vi "MULTTCP_CB_findcmd.vi"(9 "pending in":T1[](array[typedef]), 10 "message":string, 11 "cmds":string[](array[string])) -> (1 "pending out":T1[](array[typedef]), 2 "found":bool, 6 "cmd index":i32)   [LabVIEW 2016]
uses:
  MULTTCP_BlockingStruct.ctl
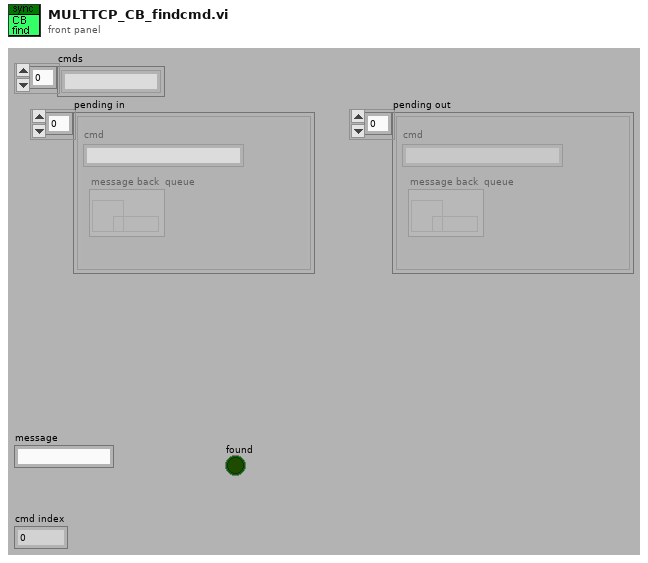
[diagram p1: front panel]
types:
  T1 = typedef "MULTTCP_BlockingStruct.ctl" = cluster{"cmd":string, "message back  queue":refnum<queue>}
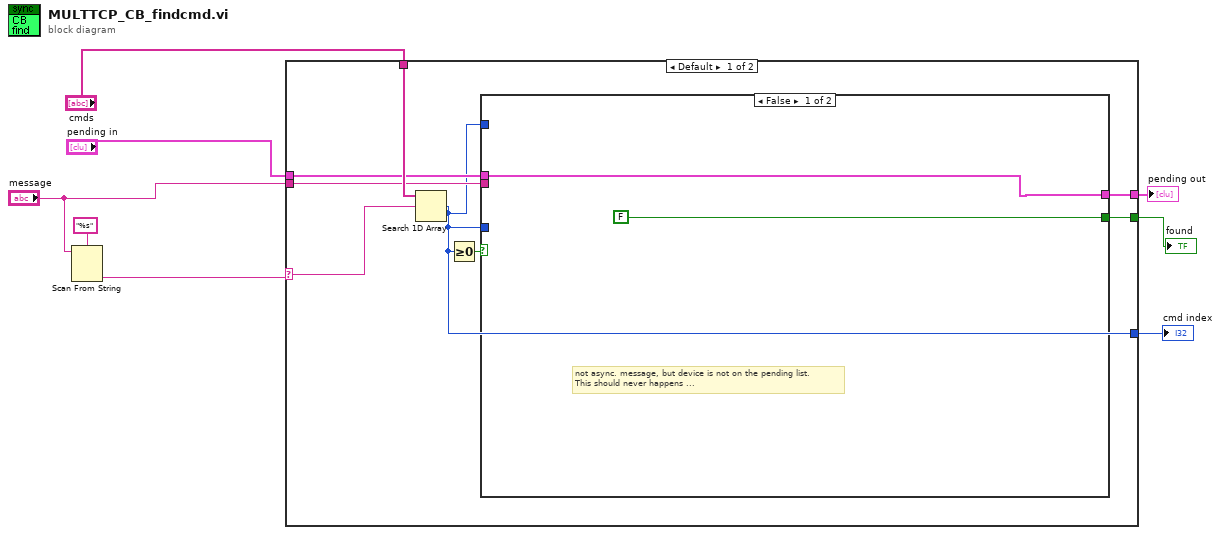
[diagram p0: block diagram]
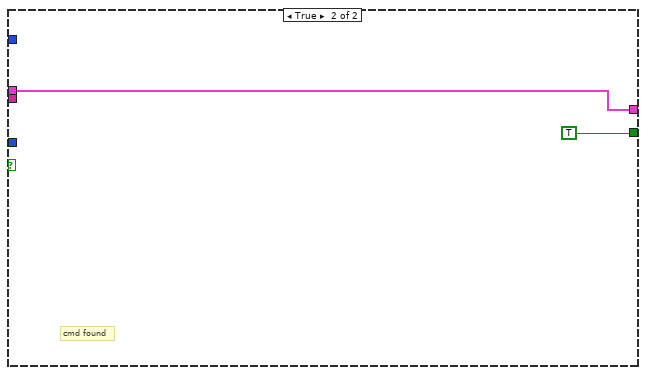
[diagram p2: hidden frame]
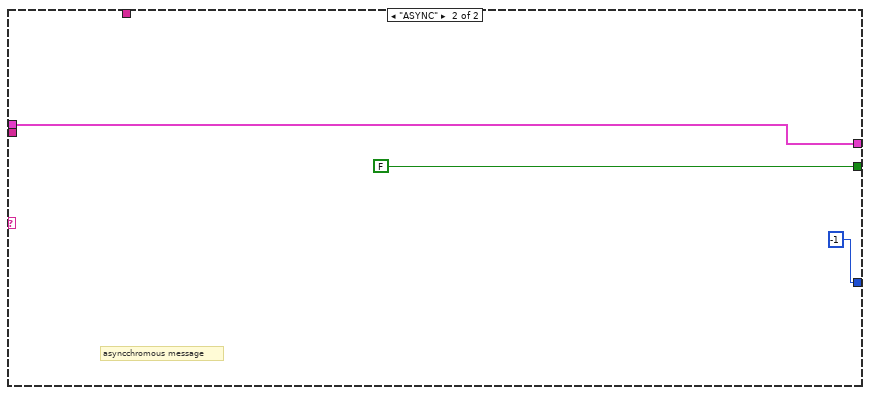
[diagram p3: hidden frame]
diagram:
  n1 = Scan From String(format string="%s", input string="message") -> (output 1=w1:string)  [unwired: 2 in, 4 out]
  n2 = case shown="Default" w1 {
    selector: w1 -> [w10 _]
    tunnel: "cmds" -> [w16 _]
    tunnel: [w14 FALSE ("status")] -> w6
    tunnel: "pending in" -> [w13 w22]
    tunnel: "message" -> [w12 _]
    tunnel: [w11 w22] -> w5
    tunnel: [w9 -1] -> w4
    frame Default {
      n3 = Search 1D Array(1D array=w16, element=w10) -> (index of element=w9:i32)  [unwired: 1 out]
      n4 = Greater Or Equal To 0?(x=w9) -> (x >= 0?=w15:bool)
      n5 = case shown="False" w15 {
        tunnel: [FALSE ("status") TRUE] -> w14
        tunnel: w13 -> [w17 w19]
        tunnel: w12 -> [_ _]
        tunnel: [w17 w19] -> w11
        tunnel: w9 -> [_ _]
        tunnel: w9 -> [_ _]
        frame False {
          # "not async. message, but device is not on the pending list.\nThis should never happens ..."
        }
        frame True {
          # "cmd found"
        }
      }
    }
    frame "ASYNC" {
      # "asyncchromous message"
    }
  }
  "found" <- w6
  "pending out" <- w5
  "cmd index" <- w4
